vi "Launch Nested.vi"(8 "Error In":errorcluster, 9 "ID":string, 10 "Nested Actor":refnum<class "Actor.lvclass">, 11 "Controller in":refnum<class "Controller.lvclass">) -> (0 "Error Out":errorcluster, 1 "Nested Actor's Enqueuer":refnum<class "Message Enqueuer.lvclass">, 2 "Launch Failure?":bool, 3 "Controller out":refnum<class "Controller.lvclass">)   [LabVIEW 2018, in "Controller.lvlib" / "Controller.lvclass"]
doc: "This VI launches the nested actor and then stores the enqueuer in a MAP object (represented by variant attributes). The enqueuer name is based on a unique <b>ID</b>. Each time an object is added, the attribute <b>NumActive</b> is incremented, the actual object (Enqueuer) is stored with a key value of <b>ID</b> and the key is added to a list of attributes called <b>IDs</b>. \n\nThe <b>NumActive</b> allows the MAP to indicate when it is empty. This is used when stopping the system.\n\nIf the launch is unsuccessful, the enqueuer is not stored and the MAP is not affected."
uses:
  Controller.lvclass
  C:/Program Files (x86)/National Instruments/LabVIEW 2018/vi.lib/ActorFramework/Actor/Actor.lvclass
  C:/Users/Labview/Documents/exscalabar_server/SuperActor/SuperActor.lvclass
  <vilib>/ActorFramework/Actor/Actor.lvclass
  <vilib>/ActorFramework/Message Enqueuer/Message Enqueuer.lvclass
  Controller.lvclass/Controller.ctl
  Controls/eMap.ctl
  SuperActor/SuperActor.lvclass/SuperActor.ctl
  SuperActor/Read Log Session.vi
  <userlib>/_Session Fwk/Session - Root.lvclass
  reusable/Session APIs/Session Log/System Log.lvclass
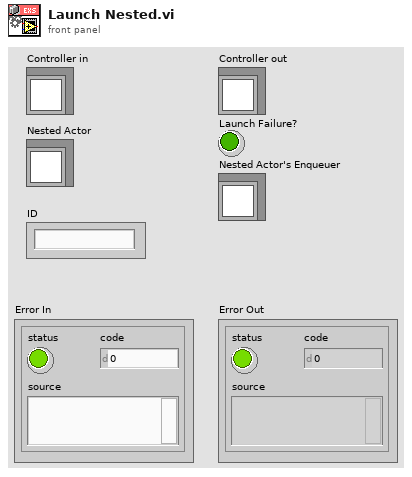
[diagram p1: front panel]
types:
  T1 = typedef "Controller.lvlib/Controller.lvclass/eMap.ctl" = cluster{"Enqueuer":refnum<class "Message Enqueuer.lvclass">, "Active":bool}
  T2 = typedef "Session - Root.lvclass/Session Handle.ctl" = refnum<data-value>
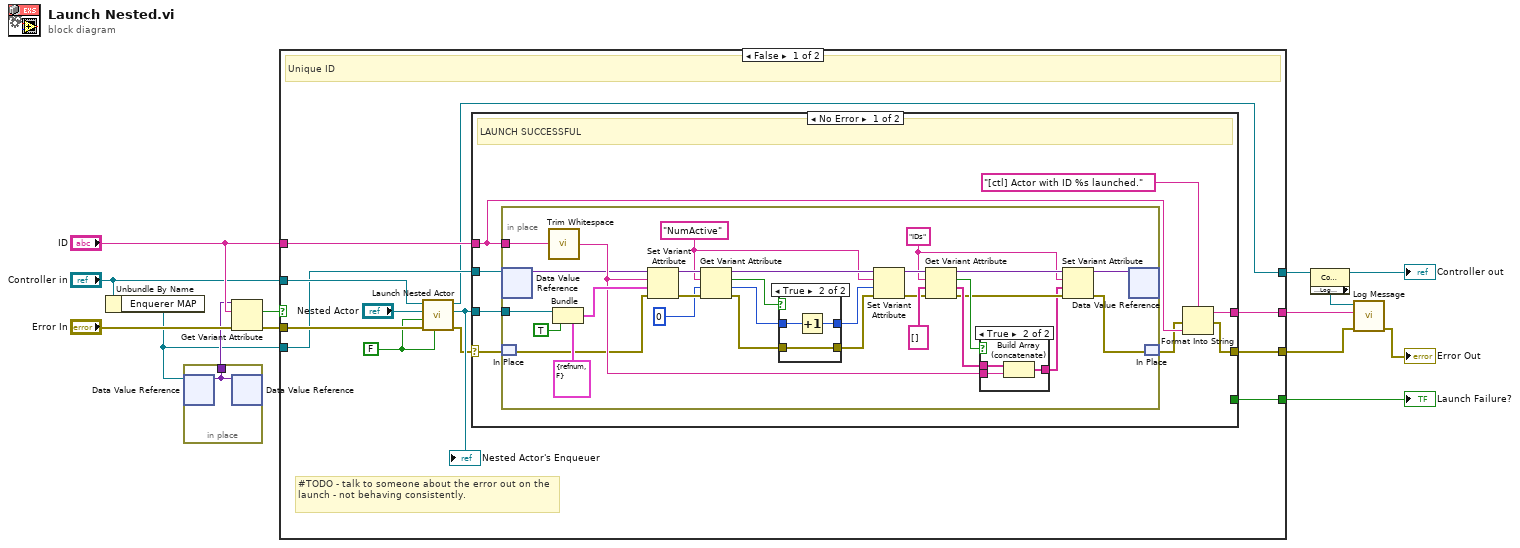
[diagram p0: block diagram]
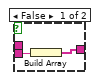
[diagram p2: hidden frame]
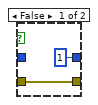
[diagram p3: hidden frame]
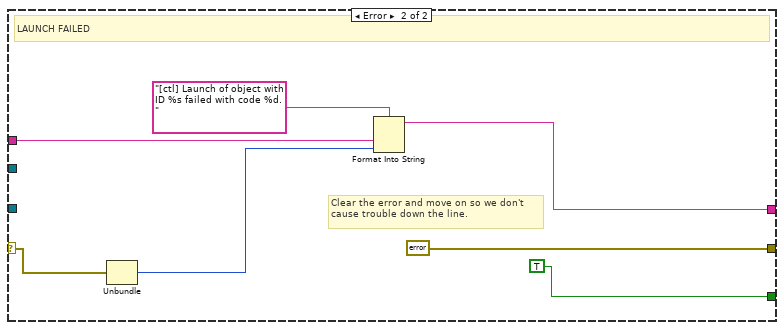
[diagram p4: hidden frame]
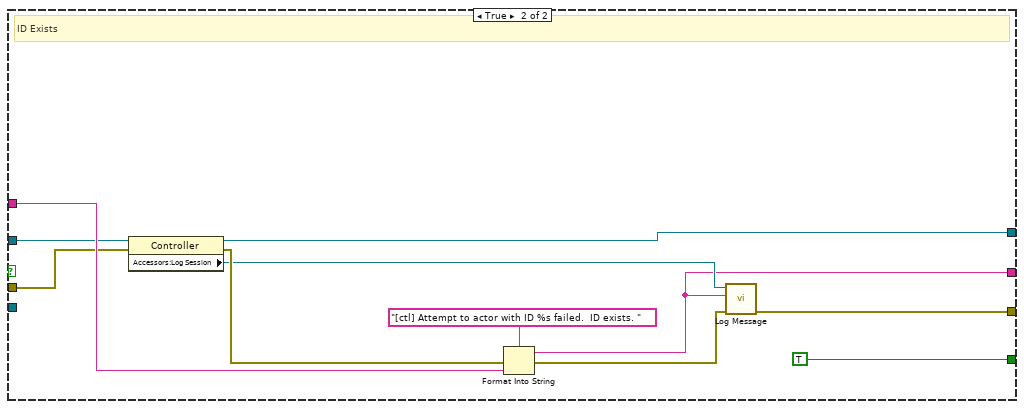
[diagram p5: hidden frame]
diagram:
  n1 = Unbundle By Name("Controller in") -> ("Enquerer MAP"=w1:refnum<data-value>)
  n2 = in-place {
    in-place-border: [w15] -> w2
    n3 = in-place-dvr #1(w1) -> (w15:variant)  [unwired: 1 out]
    n4 = in-place-dvr #1(w15) -> ()  [unwired: 2 out]
  }
  n5 = Get Variant Attribute(Variant=w2, name="ID", error in="Error In") -> (found=w11:bool, error out=w10:errorcluster)  [unwired: 1 in, 2 out]
  n6 = case shown="False" w11 {
    tunnel: "ID" -> [w25 w89]
    tunnel: [w17 w87] -> w9
    tunnel: [w24 w90] -> w6
    tunnel: "Controller in" -> [w23 w88]
    tunnel: w10 -> [w22 w85]
    tunnel: [w21 w83] -> w4
    tunnel: [w19 TRUE] -> w3
    tunnel: w1 -> [w18 _]
    frame False {
      w16 = FALSE ("Open Actor Core front panel? (F)")
      # "#TODO - talk to someone about the error out on the launch - not behaving consistently."
      # "Unique ID"
      n7 = call <vilib>:"Launch Nested Actor.vi"("Open Actor Core front panel? (F)"=w16, "error in (no error)"=w22, "Auto-stop? (T)"=w16, "Nested Actor"="Nested Actor", "Caller Actor in"=w23) -> ("error out"=w20:errorcluster, "Nested Actor's Enqueuer"=w27:refnum<class "Message Enqueuer.lvclass">, "Caller Actor out"=w17:refnum<class "Controller.lvclass">)  [unwired: 4 in]
      "Nested Actor's Enqueuer" <- w27
      n8 = case shown="No Error" w20 {
        selector: w20 -> [w34 w81]
        tunnel: w27 -> [w35 _]
        tunnel: [w28 errorcluster {"status"=FALSE, "code"=0, "source"=""} ("error IO")] -> w24
        tunnel: w25 -> [w32 w79]
        tunnel: [w31 w77] -> w21
        tunnel: [_ TRUE] -> w19
        tunnel: w18 -> [w30 _]
        frame No Error {
          # "LAUNCH SUCCESSFUL"
          n9 = in-place {
            in-place-border: w35 -> [w64]
            in-place-border: w32 -> [w41]
            w43 = "IDs" ("name")
            w53 = "NumActive" ("name")
            n10 = in-place-dvr #2(w30) -> (w37:variant)  [unwired: 1 out]
            n11 = in-place-match #3(w34) -> (w39:errorcluster)
            n12 = call <vilib>:"Trim Whitespace.vi"("string"=w41) -> ("trimmed string"=w40:string)  [unwired: 1 in]
            n13 = Bundle(cluster=T1 {"Enqueuer"=refnum, "Active"=FALSE} ("eMap"), "Enqueuer"=w64, "Active"=TRUE) -> (w63:T1)
            n14 = Set Variant Attribute(Variant=w37, name=w40, value=w63, error in=w39) -> (Variant out=w60:variant, error out=w61:errorcluster)  [unwired: 1 out]
            n15 = Get Variant Attribute(Variant=w60, name=w53, default value (empty Variant)=i16 0 ("unsigned 8bit integer"), error in=w61) -> (duplicate Variant=w57:variant, found=w56:bool, value=w59:i16, error out=w55:errorcluster)
            n16 = case shown="True" w56 {
              tunnel: w59 -> [_ w72]
              tunnel: [i16 1 w74] -> w58
              tunnel: w55 -> [w70 w73]
              tunnel: [w70 w73] -> w54
              frame False {
              }
              frame True {
                n17 = Increment(x=w72) -> (x+1=w74:i16)
              }
            }
            n18 = Set Variant Attribute(Variant=w57, name=w53, value=w58, error in=w54) -> (Variant out=w51:variant, error out=w49:errorcluster)  [unwired: 1 out]
            n19 = Get Variant Attribute(Variant=w51, name=w43, default value (empty Variant)=string[] [], error in=w49) -> (duplicate Variant=w46:variant, found=w48:bool, value=w47:string[], error out=w45:errorcluster)
            n20 = case shown="True" w48 {
              tunnel: w47 -> [_ w69]
              tunnel: w40 -> [w66 w68]
              tunnel: [w65 w67] -> w44
              frame False {
                n21 = Build Array(w66) -> (w65:string[])
              }
              frame True {
                n22 = Build Array (concatenate)(w69, w68) -> (w67:string[])
              }
            }
            n23 = Set Variant Attribute(Variant=w46, name=w43, value=w44, error in=w45) -> (Variant out=w36:variant, error out=w38:errorcluster)  [unwired: 1 out]
            n24 = in-place-dvr #2(w36) -> ()  [unwired: 2 out]
            n25 = in-place-match #3(w38) -> (w29:errorcluster)
          }
          n26 = Format Into String(format string="[ctl] Actor with ID %s launched.", error in=w29, w32) -> (resulting string=w31:string, error out=w28:errorcluster)  [unwired: 1 in]
        }
        frame Error {
          # "Clear the error and move on so we don't cause trouble down the line."
          # "LAUNCH FAILED"
          n27 = Unbundle(w81) -> ("code"=w78:i32)  [unwired: 2 out]
          n28 = Format Into String(format string="[ctl] Launch of object with ID %s failed with code %d.  ", w79, w78) -> (resulting string=w77:string)  [unwired: 2 in, 1 out]
        }
      }
    }
    frame True {
      # "ID Exists"
      n29 = property class="Controller"(reference=w88, error in=w85) -> (reference out=w87:refnum<class "Controller.lvclass">, error out=w86:errorcluster, "Accessors:Log Session"=w84:T2)
      n30 = Format Into String(format string="[ctl] Attempt to actor with ID %s failed.  ID exists. ", error in=w86, w89) -> (resulting string=w83:string, error out=w91:errorcluster)  [unwired: 1 in]
      n31 = call "Log Message.vi"("error in"=w91, "MSG In"=w83, "session in"=w84) -> ("error out"=w90:errorcluster)  [unwired: 7 in, 1 out]
    }
  }
  "Launch Failure?" <- w3
  n32 = property class="Controller"(reference=w9) -> (reference out=→"Controller out":refnum<class "Controller.lvclass">, "Accessors:Log Session"=w7:T2)  [unwired: 1 in, 1 out]
  n33 = call "Log Message.vi"("error in"=w6, "MSG In"=w4, "session in"=w7) -> ("error out"=→"Error Out":errorcluster)  [unwired: 7 in, 1 out]
